vi "Blow Air.vi"(8 "error in (no error)":errorcluster, 10 "enable?":bool, 11 "Swamp Cooler in":refnum<class "Evaporative Cooler.lvclass">) -> (0 "error out":errorcluster, 3 "Swamp Cooler out":refnum<class "Evaporative Cooler.lvclass">)   [LabVIEW 2023, in "Evaporative Cooler.lvclass"]
uses:
  Evaporative Cooler.lvclass
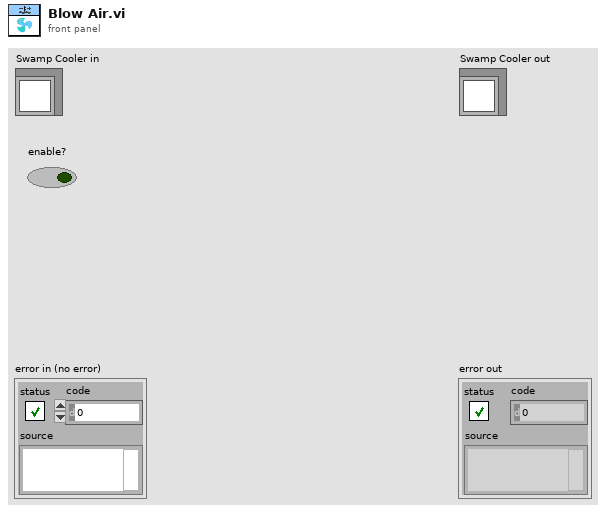
[diagram p1: front panel]
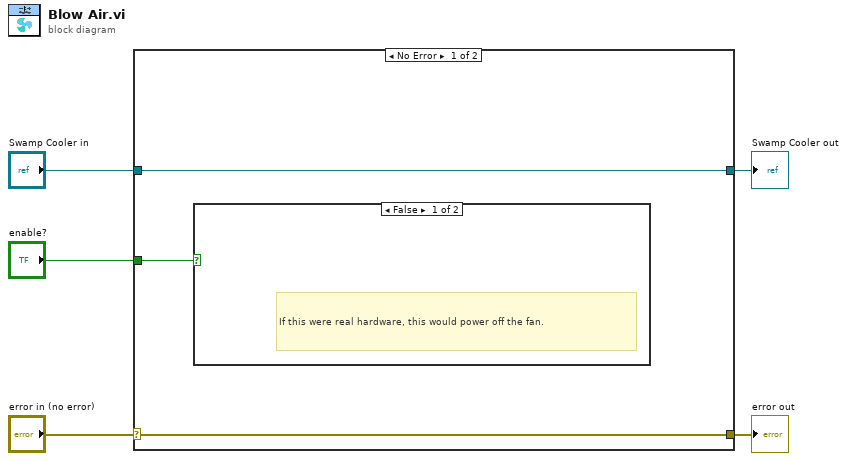
[diagram p0: block diagram]
diagram:
  n1 = case shown="No Error" "error in (no error)" {
    selector: "error in (no error)" -> [w8 w10]
    tunnel: [w8 w10] -> w4
    tunnel: [w6 w9] -> w2
    tunnel: "Swamp Cooler in" -> [w6 w9]
    tunnel: "enable?" -> [w7 _]
    frame No Error {
      n2 = case shown="False" w7 {
        frame False {
          # "If this were real hardware, this would power off the fan."
        }
        frame True {
          # "If this were real hardware, this would power on the fan."
        }
      }
    }
    frame Error {
    }
  }
  "error out" <- w4
  "Swamp Cooler out" <- w2
